vi "Get Motion Controller.vi"(8 "error in (no error)":errorcluster, 9 "Path":path, 10 "Section":string, 11 "Axis Factory in":refnum<class "Axis Factory.lvclass">) -> (0 "error out":errorcluster, 2 "iMotion Controller.lvclass":refnum<class "iMotion Controller.lvclass">, 3 "Axis Factory out":refnum<class "Axis Factory.lvclass">)   [LabVIEW 2022 SP3, in "Axis Factory.lvclass"]
uses:
  Axis Factory.lvclass
  iMotion Controller/iMotion Controller.lvclass
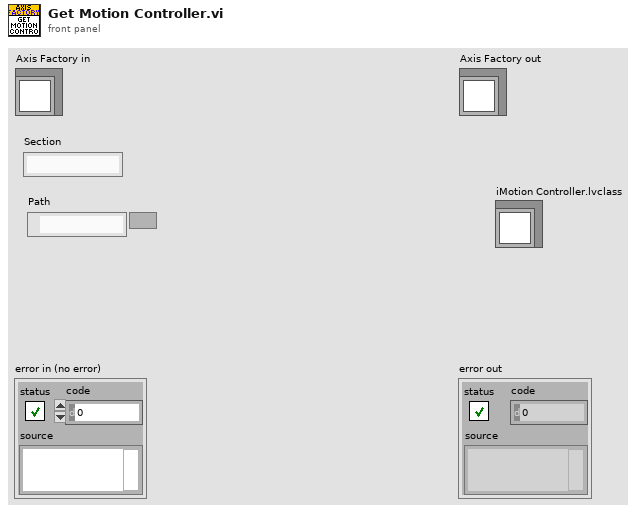
[diagram p1: front panel]
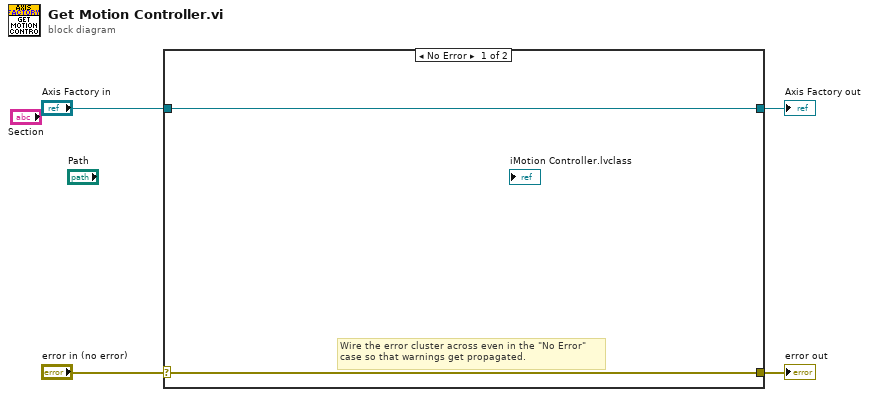
[diagram p0: block diagram]
diagram:
  n1 = case shown="No Error" "error in (no error)" {
    selector: "error in (no error)" -> [w5 w8]
    tunnel: [w5 w8] -> w3
    tunnel: [w6 w7] -> w1
    tunnel: "Axis Factory in" -> [w6 w7]
    frame No Error {
      # "Wire the error cluster across even in the \"No Error\"\ncase so that warnings get propagated."
    }
    frame Error {
    }
  }
  "error out" <- w3
  "Axis Factory out" <- w1
